vi "Get UID.vi"(8 "error in (no error)":errorcluster, 11 "Object In":refnum<class "Object.lvclass">) -> (0 "error out":errorcluster, 2 "UID":i32, 3 "Object In":refnum<class "Object.lvclass">)   [LabVIEW 2015, in "Front Panel Publisher.lvlib" / "Object.lvclass"]
uses:
  Object.lvclass
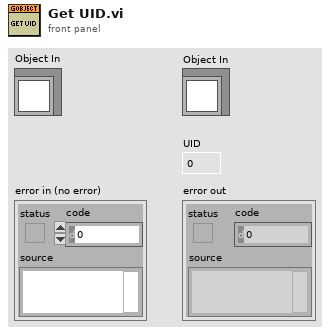
[diagram p1: front panel]
types:
  T1 = typedef "Front Panel Publisher.lvlib/Object.lvclass/Attributes.ctl" = cluster{"UID":i32, "Type":string, "Coordinates":T2, "Reference":refnum<vi>}
  T2 = typedef "Front Panel Publisher.lvlib/Object.lvclass/Coordinates.ctl" = cluster{"Left":i32, "Top":i32, "Height":u32, "Width":u32}
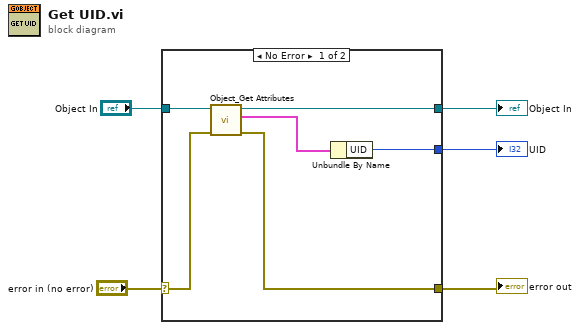
[diagram p0: block diagram]
diagram:
  n1 = case shown="No Error" "error in (no error)" {
    selector: "error in (no error)" -> [w11 w13]
    tunnel: [w9 w13] -> w4
    tunnel: [w7 w12] -> w2
    tunnel: "Object In" -> [w8 w12]
    tunnel: [w6 _] -> w1
    frame No Error {
      n2 = call "Object_Get Attributes.vi"("error in (no error)"=w11, "Object In"=w8) -> ("error out"=w9:errorcluster, "Data"=w10:T1, "Object Out"=w7:refnum<class "Object.lvclass">)  [unwired: 6 in, 1 out]
      n3 = Unbundle By Name(w10) -> ("UID"=w6:i32)
    }
    frame Error {
    }
  }
  "error out" <- w4
  "Object In" <- w2
  "UID" <- w1
